vi "GetPressure.vi"(8 "error in (no error)":errorcluster, 11 "GenericPG in":refnum<class "GenericPG.lvclass">) -> (0 "error out":errorcluster, 2 "Pressure (mbar)":dbl, 3 "GenericPG out":refnum<class "GenericPG.lvclass">)   [LabVIEW 2016, in "GenericPG.lvlib" / "GenericPG.lvclass"]
uses:
  GenericPG.lvclass
  GenericPG.lvclass/GenericPG.ctl
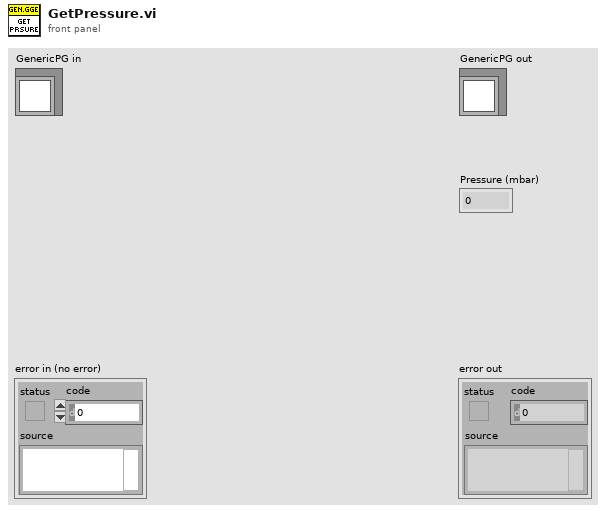
[diagram p1: front panel]
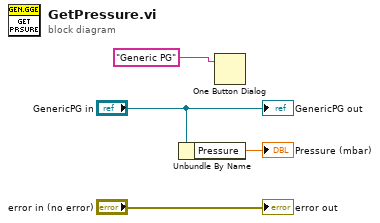
[diagram p0: block diagram]
diagram:
  n1 = Unbundle By Name("GenericPG in") -> ("Pressure"=→"Pressure (mbar)":dbl)
  n2 = One Button Dialog(message="Generic PG" ("button name (\"OK\")")) -> ()  [unwired: 1 in, 1 out]
  "error out" <- "error in (no error)"
  "GenericPG out" <- "GenericPG in"
